vi "value_within_range.vi"(9 "Error range":dbl, 10 "Target Value":dbl, 11 "Actual Value":dbl) -> (3 "within_range?":bool)   [LabVIEW 2020]
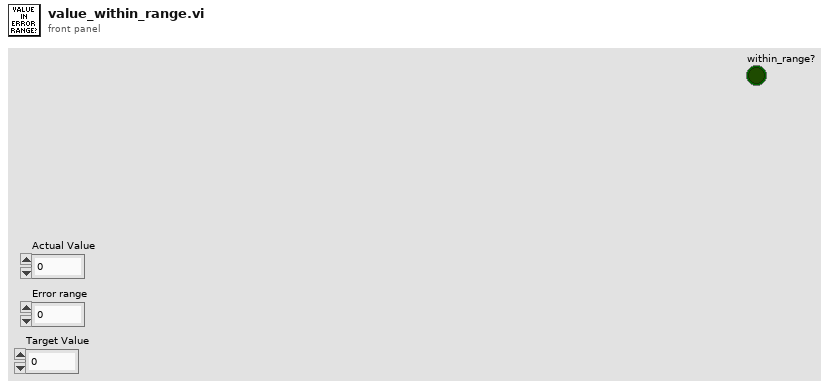
[diagram p1: front panel]
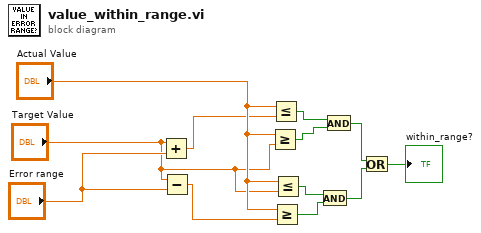
[diagram p0: block diagram]
diagram:
  n1 = Add(x="Target Value", y="Error range") -> (x+y=w8:dbl)
  n2 = Subtract(x="Target Value", y="Error range") -> (x-y=w10:dbl)
  n3 = Greater Or Equal?(x="Actual Value", y="Target Value") -> (x >= y?=w6:bool)
  n4 = Less Or Equal?(x="Actual Value", y=w8) -> (x <= y?=w7:bool)
  n5 = Greater Or Equal?(x="Actual Value", y=w10) -> (x >= y?=w4:bool)
  n6 = Less Or Equal?(x="Actual Value", y="Target Value") -> (x <= y?=w5:bool)
  n7 = And(x=w5, y=w4) -> (x .and. y?=w2:bool)
  n8 = And(x=w7, y=w6) -> (x .and. y?=w3:bool)
  n9 = Or(x=w3, y=w2) -> (x .or. y?=→"within_range?":bool)
